vi "DATA_Reorder_after_condition_modification.vi"(3 "Array of conditions":T8 {"Specifier(s)"."Validity criteria(s)"."Validity value" min=0.0 step=0.1 format="%.2g"; "Specifier(s)"."Value" step=1.0 format="%#.2g"}) -> (1 "Reordered conditions array":T1[](array[typedef]) {"Specifier(s)"."Validity criteria(s)"."Validity value" min=0.0 step=0.1 format="%.2g"; "Specifier(s)"."Value" step=1.0 format="%#.2g"})   [LabVIEW 2018, in "Tracker.lvlib"]
uses:
  Tracker.lvlib
  Controls/CTL_Conditions_Array.ctl
  Controls/CTL_Conditions_Cluster.ctl
  Controls/CTL_Condition_type.ctl
  Controls/CTL_Comparison_type.ctl
  Controls/CTL_Validity_check_criteria.ctl
  Controls/CTL_Response_info.ctl
  Controls/CTL_Condition_response_type.ctl
  Controls/CTL_Reponse_port_info.ctl
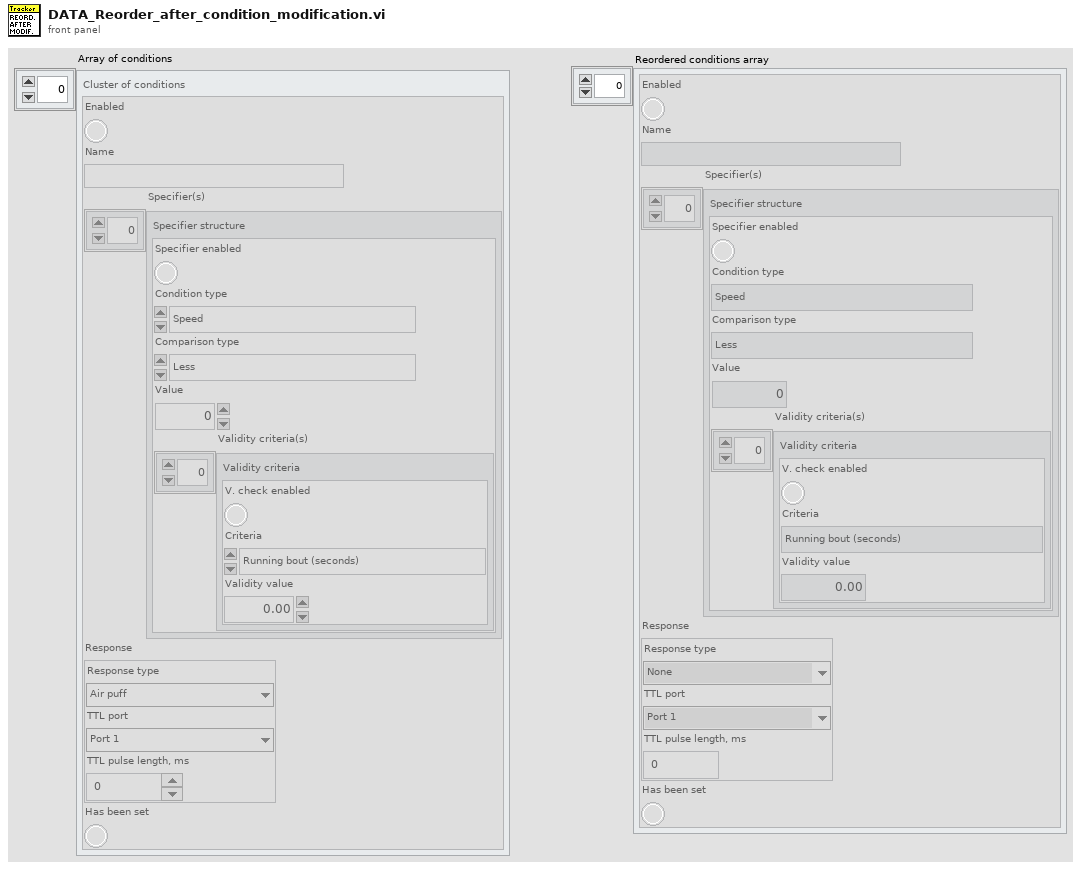
[diagram p1: front panel]
types:
  T1 = typedef "Tracker.lvlib/CTL_Conditions_Cluster.ctl" = cluster{"Enabled":bool, "Name":string, "Specifier(s)":cluster{"Specifier enabled":bool, "Condition type":T2, "Comparison type":T3, "Value":dbl, "Validity criteria(s)":cluster{"V. check enabled":bool, "Criteria":T4, "Validity value":dbl}[]}[], "Response":T5, "Has been set":bool}
  T2 = typedef "Tracker.lvlib/CTL_Condition_type.ctl" = enum16{"Speed", "Zone", "Angle to wall"}
  T3 = typedef "Tracker.lvlib/CTL_Comparison_type.ctl" = enum16{"Less", "Less or Equal", "Equal", "Greater or Equal", "Greater", "Not Equal"}
  T4 = typedef "Tracker.lvlib/CTL_Validity_check_criteria.ctl" = enum16{"Running bout (seconds)", "Running bout (meters)"}
  T5 = typedef "Tracker.lvlib/CTL_Response_info.ctl" = cluster{"Response type":T6, "TTL port":T7, "TTL pulse length, ms":dbl}
  T6 = typedef "Tracker.lvlib/CTL_Condition_response_type.ctl" = enum16{"None", "Air puff", "Liquid reward"}
  T7 = typedef "Tracker.lvlib/CTL_Reponse_port_info.ctl" = enum16{"Port 1", "Port 2", "Port 3", "Port 4"}
  T8 = typedef "Tracker.lvlib/CTL_Conditions_Array.ctl" = T1[]
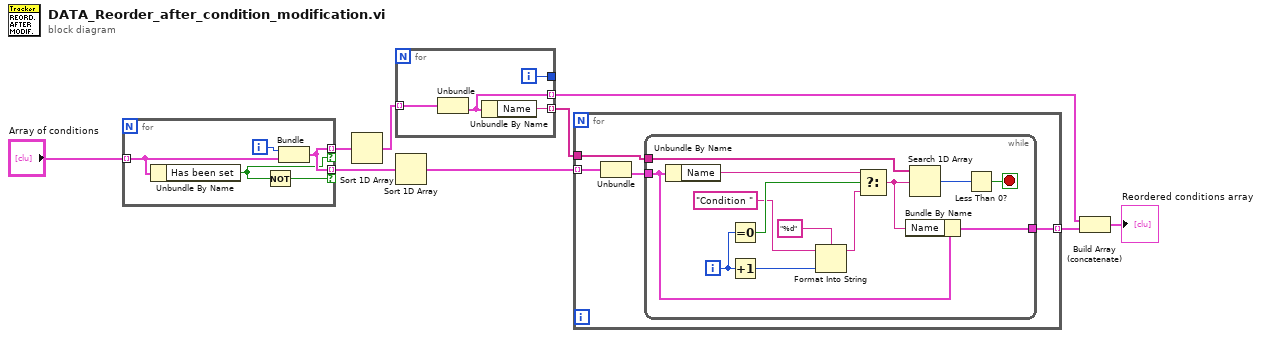
[diagram p0: block diagram]
diagram:
  n1 = for {
    tunnel: "Array of conditions" -> [w13] mode=indexing
    tunnel: [w12] -> w8 mode=indexing if=w11
    tunnel: [w12] -> w7 mode=indexing if=w10
    i -> [w14]
    n2 = Unbundle By Name(w13) -> ("Has been set"=w11:bool)
    n3 = Not(x=w11) -> (.not. x?=w10:bool)
    n4 = Bundle(w14, "Cluster of conditions"=w13) -> (w12:cluster{i32, "Cluster of conditions":T1})  [unwired: 1 in]
  }
  n5 = Sort 1D Array(array=w8) -> (sorted array=w6:cluster{i32, "Cluster of conditions":T1}[])
  n6 = for {
    tunnel: w6 -> [w18] mode=indexing
    tunnel: [w16] -> w2 mode=indexing
    tunnel: [w17] -> _
    tunnel: [w15] -> w1 mode=indexing
    i -> [w17]
    n7 = Unbundle(w18) -> ("Cluster of conditions"=w16:T1)  [unwired: 1 out]
    n8 = Unbundle By Name(w16) -> ("Name"=w15:string)
  }
  n9 = Sort 1D Array(array=w7) -> (sorted array=w5:cluster{i32, "Cluster of conditions":T1}[])
  n10 = for {
    tunnel: w5 -> [w22] mode=indexing
    tunnel: [w19] -> w4 mode=indexing
    tunnel: w1 -> [w21]
    n11 = Unbundle(w22) -> ("Cluster of conditions"=w20:T1)  [unwired: 1 out]
    n12 = while {
      tunnel: w21 -> [w34]
      tunnel: w20 -> [w25]
      tunnel: [w23] -> w19
      i -> [w27]
      stop <- w33 stop-if-true
      n13 = Unbundle By Name(w25) -> ("Name"=w31:string)
      n14 = Equal To 0?(x=w27) -> (x = 0?=w32:bool)
      n15 = Increment(x=w27) -> (x+1=w30:i32)
      n16 = Format Into String(format string="%d", initial string="Condition ", w30) -> (resulting string=w26:string)  [unwired: 1 in, 1 out]
      n17 = Select(t=w31, s=w32, f=w26) -> (s? t:f=w24:string)
      n18 = Bundle By Name(cluster=w25, "Name"=w24) -> (w23:T1)
      n19 = Search 1D Array(1D array=w34, element=w24) -> (index of element=w35:i32)  [unwired: 1 in]
      n20 = Less Than 0?(x=w35) -> (x < 0?=w33:bool)
    }
  }
  n21 = Build Array (concatenate)(w2, w4) -> (→"Reordered conditions array":T1[])
